vi "Get Plot Data.vi"(6 "Index":i32, 7 "2D Plot Datatype.lvclass in":refnum<class "2D Plot Datatype.lvclass">, 8 "error in (no error)":errorcluster, 10 "Multiplot Representation In":T1) -> (0 "error out":errorcluster, 2 "Multiplot Representation Out":T1, 5 "2D Plot Datatype.lvclass out":refnum<class "2D Plot Datatype.lvclass">)   [LabVIEW 2020, in "2D Plot Datatype.lvclass"]
uses:
  <vilib>/Math Plots/2D Math Plots/2D Plot/2D Plot Datatype/2D Plot Datatype.lvclass
  <vilib>/Math Plots/2D Math Plots/2D Plot/2D Plot/Typedef/Multiplot Representation.ctl
  <vilib>/Math Plots/2D Math Plots/2D Plot/2D Plot/Typedef/Plot Representation.ctl
  <vilib>/Math Plots/2D Math Plots/2D Plot/2D Plot/Typedef/Range Cluster.ctl
  <vilib>/Math Plots/2D Math Plots/2D Plot/2D Plot/2D Plot.lvclass
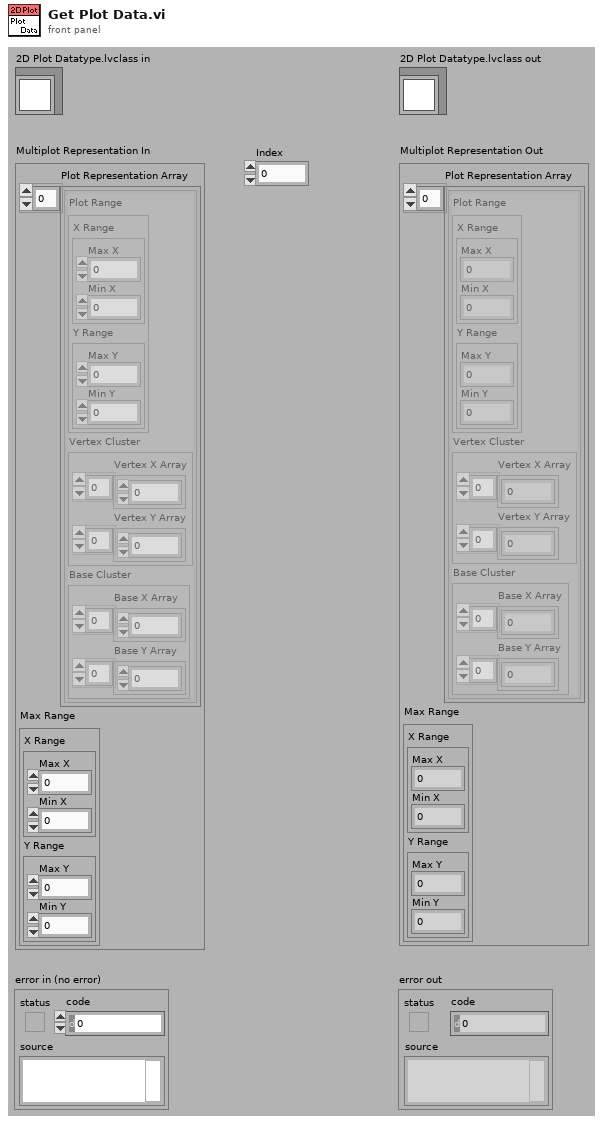
[diagram p1: front panel]
types:
  T1 = typedef "2D Plot.lvclass/Multiplot Representation.ctl" = cluster{"Plot Representation Array":T2[], "Max Range":T3}
  T2 = typedef "2D Plot.lvclass/Plot Representation.ctl" = cluster{"Plot Range":T3, "Vertex Cluster":cluster{"Vertex X Array":dbl[], "Vertex Y Array":dbl[]}, "Base Cluster":cluster{"Base X Array":dbl[], "Base Y Array":dbl[]}}
  T3 = typedef "2D Plot.lvclass/Range Cluster.ctl" = cluster{"X Range":cluster{"Max X":dbl, "Min X":dbl}, "Y Range":cluster{"Max Y":dbl, "Min Y":dbl}}
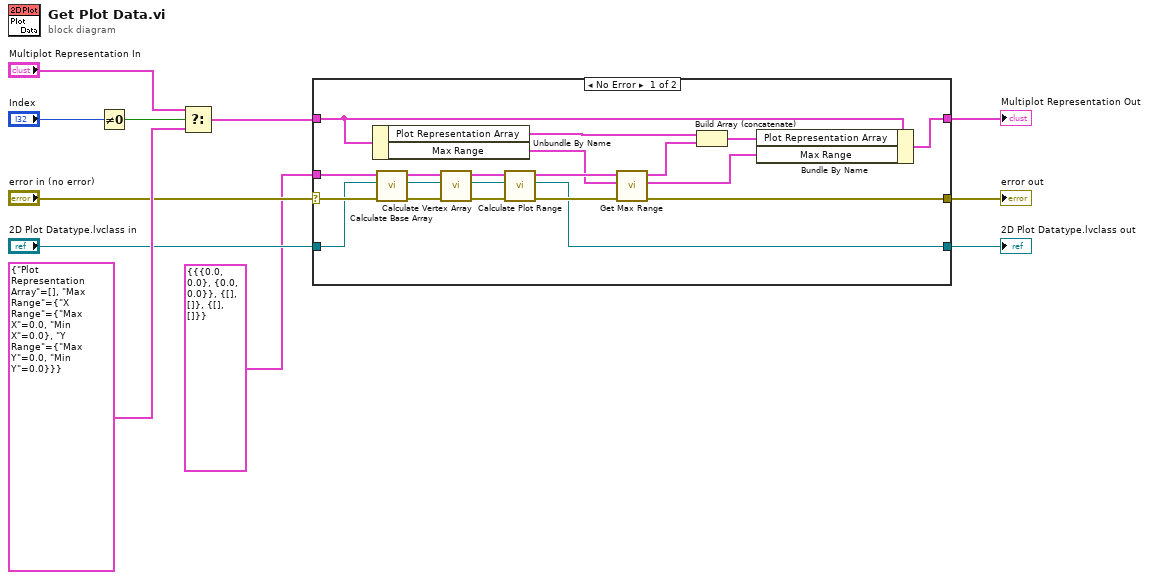
[diagram p0: block diagram]
diagram:
  n1 = Not Equal To 0?(x="Index") -> (x != 0?=w11:bool)
  n2 = Select(t="Multiplot Representation In", s=w11, f=T1 {"Plot Representation Array"=[], "Max Range"={"X Range"={"Max X"=0.0, "Min X"=0.0}, "Y Range"={"Max Y"=0.0, "Min Y"=0.0}}} ("Multiplot Representation In")) -> (s? t:f=w7:T1)
  n3 = case shown="No Error" "error in (no error)" {
    selector: "error in (no error)" -> [w14 w33]
    tunnel: w7 -> [w30 w34]
    tunnel: [w28 w34] -> w6
    tunnel: "2D Plot Datatype.lvclass in" -> [w13 w32]
    tunnel: [w22 w33] -> w5
    tunnel: [w21 w32] -> w3
    tunnel: T2 {"Plot Range"={"X Range"={"Max X"=0.0, "Min X"=0.0}, "Y Range"={"Max Y"=0.0, "Min Y"=0.0}}, "Vertex Cluster"={"Vertex X Array"=[], "Vertex Y Array"=[]}, "Base Cluster"={"Base X Array"=[], "Base Y Array"=[]}} ("Plot Representation") -> [w12 _]
    frame No Error {
      n4 = Unbundle By Name(w30) -> ("Plot Representation Array"=w31:T2[], "Max Range"=w26:T3)
      n5 = call-dynamic "Calculate Base Array.vi"("error in (no error)"=w14, "2D Plot Datatype.lvclass in"=w13, "Plot Representation In"=w12) -> ("error out"=w15:errorcluster, "2D Plot Datatype.lvclass out"=w16:refnum<class "2D Plot Datatype.lvclass">, "Plot Representation Out"=w17:T2)  [unwired: 6 out]
      n6 = call-dynamic "Calculate Vertex Array.vi"("error in (no error)"=w15, "2D Plot Datatype.lvclass in"=w16, "Plot Representation In"=w17) -> ("error out"=w18:errorcluster, "2D Plot Datatype.lvclass out"=w19:refnum<class "2D Plot Datatype.lvclass">, "Plot Representation Out"=w20:T2)  [unwired: 6 out]
      n7 = call-dynamic "Calculate Plot Range.vi"("error in (no error)"=w18, "2D Plot Datatype.lvclass in"=w19, "Plot Representation In"=w20) -> ("error out"=w23:errorcluster, "2D Plot Datatype.lvclass out"=w21:refnum<class "2D Plot Datatype.lvclass">, "Plot Representation Out"=w27:T2)  [unwired: 6 out]
      n8 = call <vilib>:"Get Max Range.vi"("error in (no error)"=w23, "Max Range In"=w26, "Plot Representation In"=w27) -> ("error out"=w22:errorcluster, "Max Range Out"=w24:T3, "Plot Representation Out"=w25:T2)  [unwired: 6 out]
      n9 = Build Array (concatenate)(w31, w25) -> (w29:T2[])
      n10 = Bundle By Name(cluster=w30, "Plot Representation Array"=w29, "Max Range"=w24) -> (w28:T1)
    }
    frame Error {
    }
  }
  "2D Plot Datatype.lvclass out" <- w3
  "Multiplot Representation Out" <- w6
  "error out" <- w5
